vi "Operation_1600X900.vi"() -> ()   [LabVIEW 2015]
uses:
  Global/Globalclient.vi
panel:
  in  "F 4":bool
  in  "F 3":bool
  in  "F 2":bool
  in  "F 1":bool
  in  "Stop Button":bool
  out "删除通道":string[](array[string])
  out "选中行":i32
  in  "Tab":enum32{"用户管理", "通道控制", "通道监测", "温度&风扇"}(tab)=enum."通道控制"
  out "连接数":u8
  out "未登陆":string[][](table)=[["admin", "123456", "ADMIN"], ["api1", "333333", "API"], ["api2", "333333", "API"], ["api3", "333333", "API"], ["weily", "123", "GENERAL"]]
  out "已登陆":string[][](table)
  in  "Add Button":bool
  in  "Remove Button":bool
  out "删除用户":string
  out "时钟":string[][](table)
  out "射频":string[][](table)
  in  "查询开关":bool
  in  "释放所有":bool
  out "LOSS":cluster{dbl[], dbl[]}[](graph)
  in  "申请通道":bool
  in  "释放通道":bool
  in  "查询差损":bool
  in  "通道":i32[](listbox)
  in  "Tab":enum32{"RF", "CLK"}(tab)
  in  "监控":enum32{"RF", "TIME"}(tab)
  out "b 1":bool
  out "b 2":bool
  out "b 3":bool
  out "b 4":bool
  out "b 5":bool
  out "b 6":bool
  out "b 7":bool
  out "b 8":bool
  out "b 9":bool
  out "b 10":bool
  out "b 11":bool
  out "b 12":bool
  out "b 13":bool
  out "b 14":bool
  out "b 15":bool
  out "b 16":bool
  out "b 17":bool
  out "b 18":bool
  out "b 19":bool
  out "b 20":bool
  out "b 21":bool
  out "b 22":bool
  out "b 23":bool
  out "b 24":bool
  out "b 25":bool
  out "b 26":bool
  out "b 27":bool
  out "b 28":bool
  out "b 29":bool
  out "b 30":bool
  out "b 31":bool
  out "b 32":bool
  out "S 1":string
  out "S 2":string
  out "S 3":string
  out "S 4":string
  out "S 5":string
  out "S 6":string
  out "S 7":string
  out "S 8":string
  out "S 9":string
  out "S 10":string
  out "S 11":string
  out "S 12":string
  out "S 13":string
  out "S 14":string
  out "S 15":string
  out "S 16":string
  out "S 17":string
  out "S 18":string
  out "S 19":string
  out "S 20":string
  out "S 21":string
  out "S 22":string
  out "S 23":string
  out "S 24":string
  out "S 25":string
  out "S 26":string
  out "S 27":string
  out "S 28":string
  out "S 29":string
  out "S 30":string
  out "S 31":string
  out "S 32":string
  out "b 33":bool
  out "b 41":bool
  out "b 49":bool
  out "b 57":bool
  out "S 33":string
  out "S 41":string
  out "S 49":string
  out "S 57":string
  out "a 9":bool
  out "b 34":bool
  out "b 42":bool
  out "b 50":bool
  out "b 58":bool
  out "S 34":string
  out "S 42":string
  out "S 50":string
  out "S 58":string
  out "a 10":bool
  out "b 35":bool
  out "b 43":bool
  out "b 51":bool
  out "b 59":bool
  out "S 35":string
  out "S 43":string
  out "S 51":string
  out "S 59":string
  out "a 11":bool
  out "b 36":bool
  out "b 44":bool
  out "b 52":bool
  out "b 60":bool
  out "S 36":string
  out "S 44":string
  out "S 52":string
  out "S 60":string
  out "a 12":bool
  out "b 37":bool
  out "b 45":bool
  out "b 53":bool
  out "b 61":bool
  out "S 37":string
  out "S 45":string
  out "S 53":string
  out "S 61":string
  out "a 13":bool
  out "b 38":bool
  out "b 46":bool
  out "b 54":bool
  out "b 62":bool
  out "S 38":string
  out "S 46":string
  out "S 54":string
  out "S 62":string
  out "a 14":bool
  out "b 39":bool
  out "b 47":bool
  out "b 55":bool
  out "b 63":bool
  out "S 39":string
  out "S 47":string
  out "S 55":string
  out "S 63":string
  out "a 15":bool
  out "b 40":bool
  out "b 48":bool
  out "b 56":bool
  out "b 64":bool
  out "S 40":string
  out "S 48":string
  out "S 56":string
  out "S 64":string
  out "a 16":bool
  out "A 9":bool
  out "A 16":bool
  out "A 15":bool
  out "A 14":bool
  out "A 13":bool
  out "A 12":bool
  out "A 11":bool
  out "A 10":bool
  out "A 1":bool
  out "a 1":bool
  out "a 2":bool
  out "A 2":bool
  out "a 3":bool
  out "A 3":bool
  out "a 4":bool
  out "A 4":bool
  out "a 5":bool
  out "A 5":bool
  out "a 6":bool
  out "A 6":bool
  out "a 7":bool
  out "A 7":bool
  out "a 8":bool
  out "A 8":bool
  out "COM 1":bool
  out "com_1":bool
  out "com_2":bool
  out "COM 2":bool
  out "com_3":bool
  out "COM 3":bool
  out "com_4":bool
  out "COM 4":bool
  out "T 1":bool caption="1"
  out "T 2":bool caption="2"
  out "T 3":bool caption="3"
  out "T 4":bool caption="4"
  out "T 5":bool caption="5"
  out "T 6":bool caption="6"
  out "T 7":bool caption="7"
  out "T 8":bool caption="8"
  out "T 9":bool caption="9"
  out "T 10":bool caption="10"
  out "T 11":bool caption="11"
  out "T 12":bool caption="12"
  out "T 13":bool caption="13"
  out "T 14":bool caption="14"
  out "T 15":bool caption="15"
  out "T 16":bool caption="16"
  out "T 17":bool caption="17"
  out "T 18":bool caption="18"
  out "T 19":bool caption="19"
  out "T 20":bool caption="20"
  out "T 21":bool caption="21"
  out "T 22":bool caption="22"
  out "T 23":bool caption="23"
  out "T 24":bool caption="24"
  out "T 25":bool caption="25"
  out "T 26":bool caption="26"
  out "T 27":bool caption="27"
  out "T 28":bool caption="28"
  out "T 29":bool caption="29"
  out "T 30":bool caption="30"
  out "T 31":bool caption="31"
  out "T 32":bool caption="32"
  out "T 33":bool caption="33"
  out "T 34":bool caption="34"
  out "T 35":bool caption="35"
  out "T 36":bool caption="36"
  out "T 37":bool caption="37"
  out "T 38":bool caption="38"
  out "T 39":bool caption="39"
  out "T 40":bool caption="40"
  out "T 41":bool caption="41"
  out "T 42":bool caption="42"
  out "T 43":bool caption="43"
  out "T 44":bool caption="44"
  out "T 45":bool caption="45"
  out "T 46":bool caption="46"
  out "T 47":bool caption="47"
  out "T 48":bool caption="48"
  out "OUT 1":bool
  out "OUT 2":bool
  out "OUT 4":bool
  out "OUT 3":bool
  out "OUT 5":bool
  out "OUT 6":bool
  out "OUT 8":bool
  out "OUT 7":bool
  in  "Alarm":bool
  in  "风扇 4":string
  out "FS 4":u16(ring)
  in  "风扇 3":string
  out "FS 3":u16(ring)
  in  "风扇 2":string
  out "FS 2":u16(ring)
  in  "风扇 1":string
  out "FS 1":u16(ring)
  out "温度 8":dbl(slide)=50.0 scale=0.0..100.0 scale format="%0.1f"
  out "温度 7":dbl(slide)=50.0 scale=0.0..100.0 scale format="%0.1f"
  out "温度 6":dbl(slide)=50.0 scale=0.0..100.0 scale format="%0.1f"
  out "温度 5":dbl(slide)=50.0 scale=0.0..100.0 scale format="%0.1f"
  out "温度 4":dbl(slide)=50.0 scale=0.0..100.0 scale format="%0.1f"
  out "温度 3":dbl(slide)=50.0 scale=0.0..100.0 scale format="%0.1f"
  out "温度 2":dbl(slide)=50.0 scale=0.0..100.0 scale format="%0.1f"
  out "温度 1":dbl(slide)=50.0 scale=0.0..100.0 scale format="%0.1f"
  in  "机箱":T1(tab)
  # "LCBB多路开关矩阵"
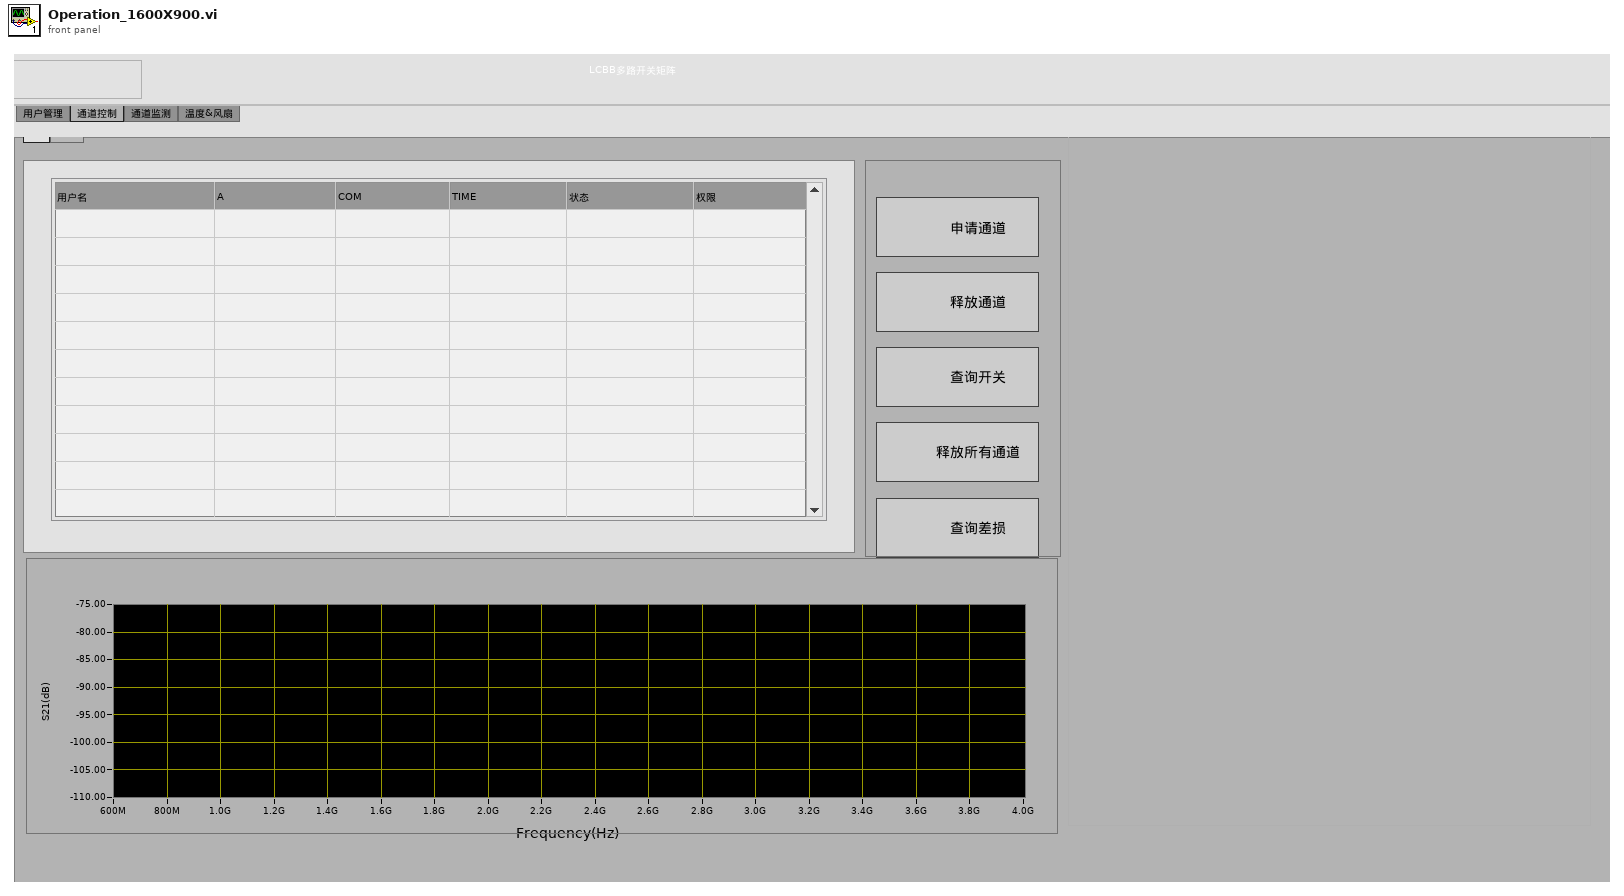
[diagram p1: front panel]
types:
  T1 = enum32{"机箱 1", "机箱 2", "机箱 3", "机箱 4", "机箱 5", "机箱 6", "机箱 7", "机箱 8", "主控 1", "机箱 9", "机箱 10", "机箱 11", "机箱 12", "机箱 13", "机箱 14", "机箱 15", "机箱 16", "主控 2"}
  T2 = enum16{"Standard", "Buffered", "CRLF", "Immediate"}
  T3 = typedef "LVPoint32TypeDef.ctl" = cluster{"Horizontal":i32, "Vertical":i32}
  T4 = typedef "LVRowAndColumnTypeDef.ctl" = cluster{"Row":i32, "Column":i32}
  T5 = cluster{"data name":string, "data data":string}[]
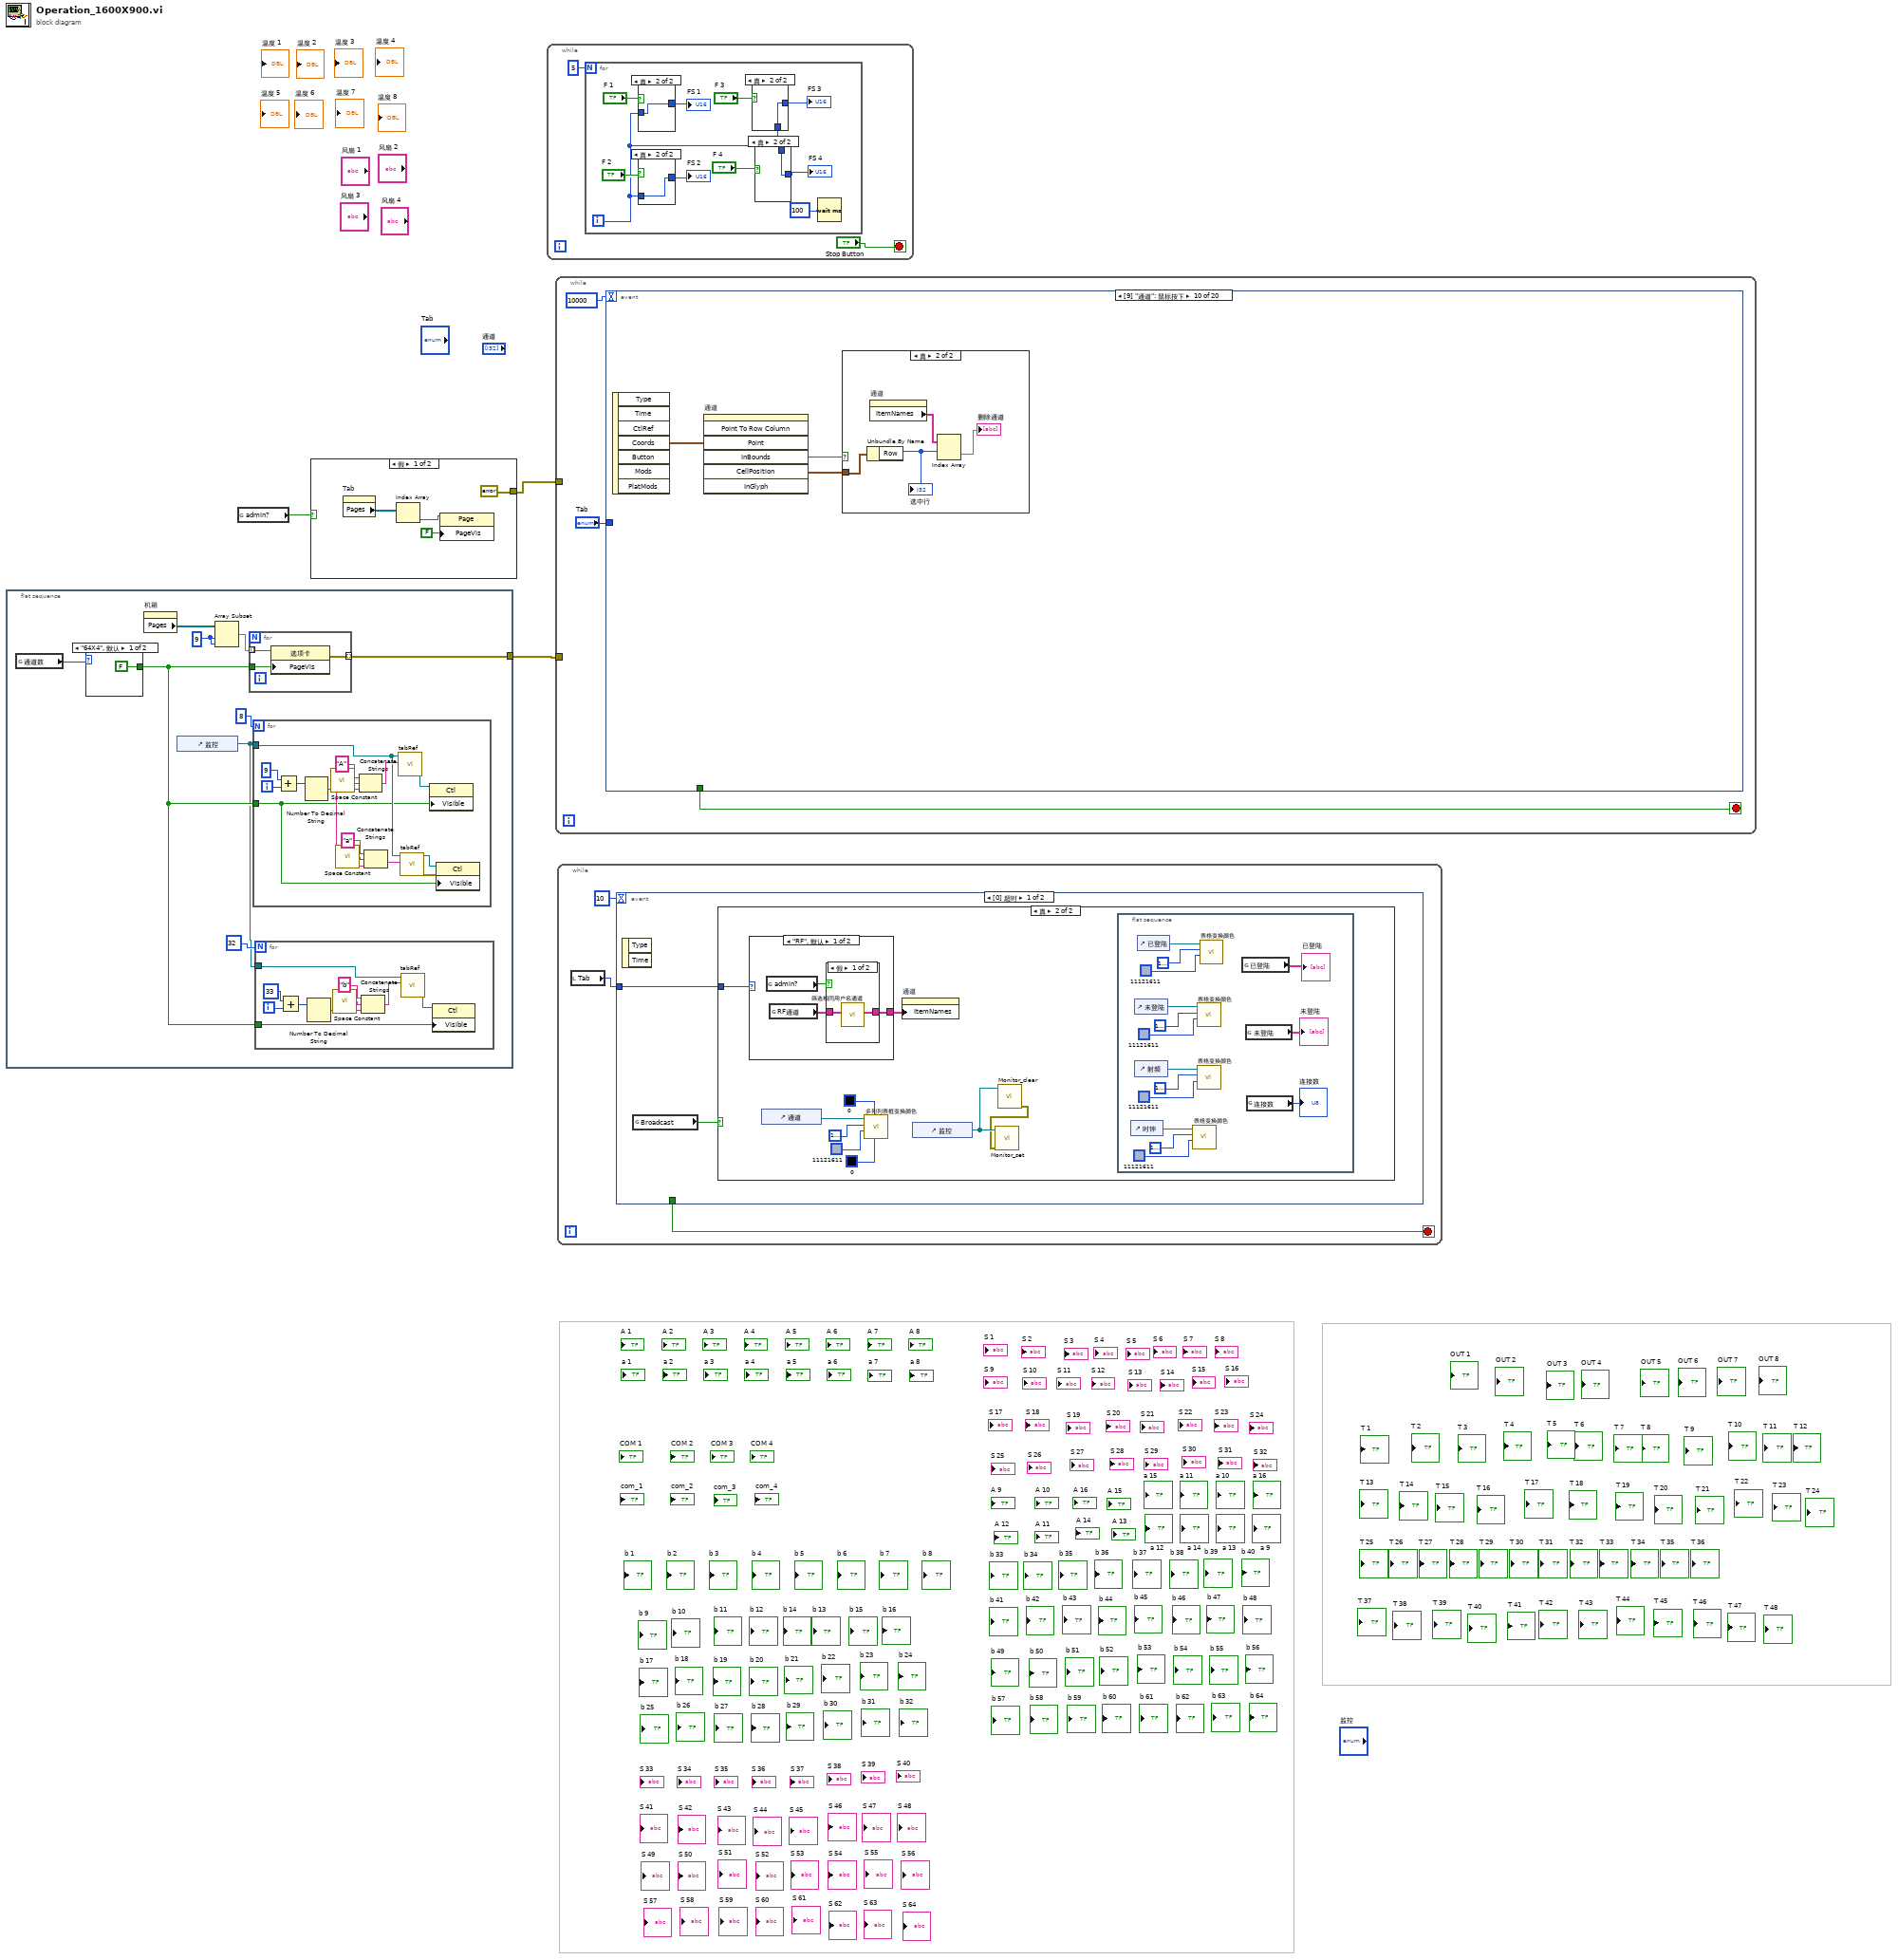
[diagram p0: block diagram]
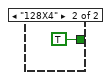
[diagram p2: hidden frame]
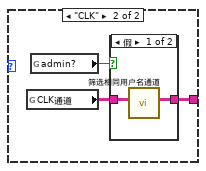
[diagram p5: hidden frame]
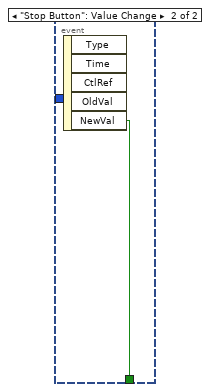
[diagram p7: hidden frame]
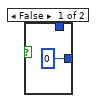
[diagram p8: hidden frame]
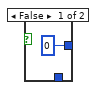
[diagram p9: hidden frame]
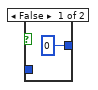
[diagram p10: hidden frame]
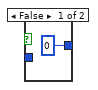
[diagram p11: hidden frame]
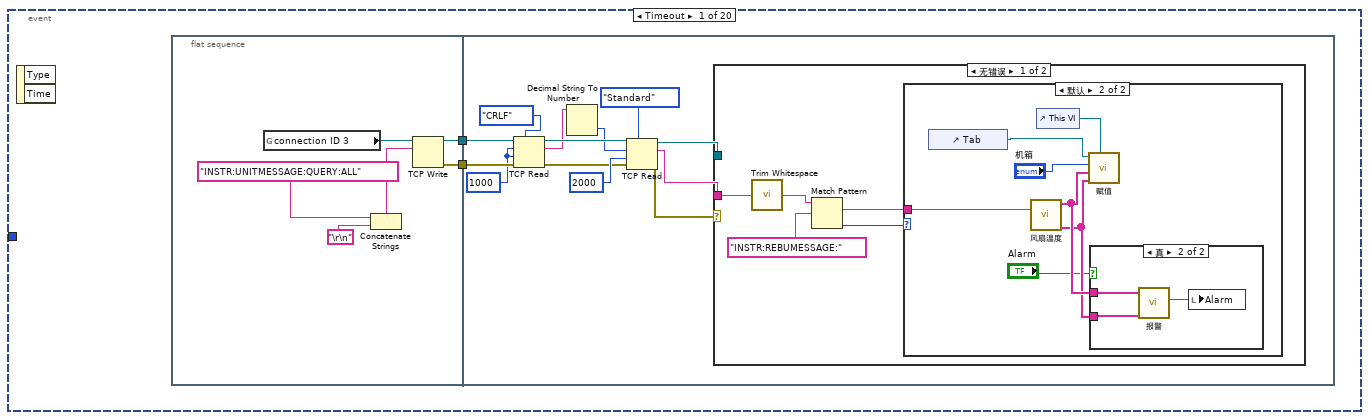
[diagram p13: hidden frame]
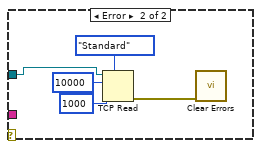
[diagram p16: hidden frame]
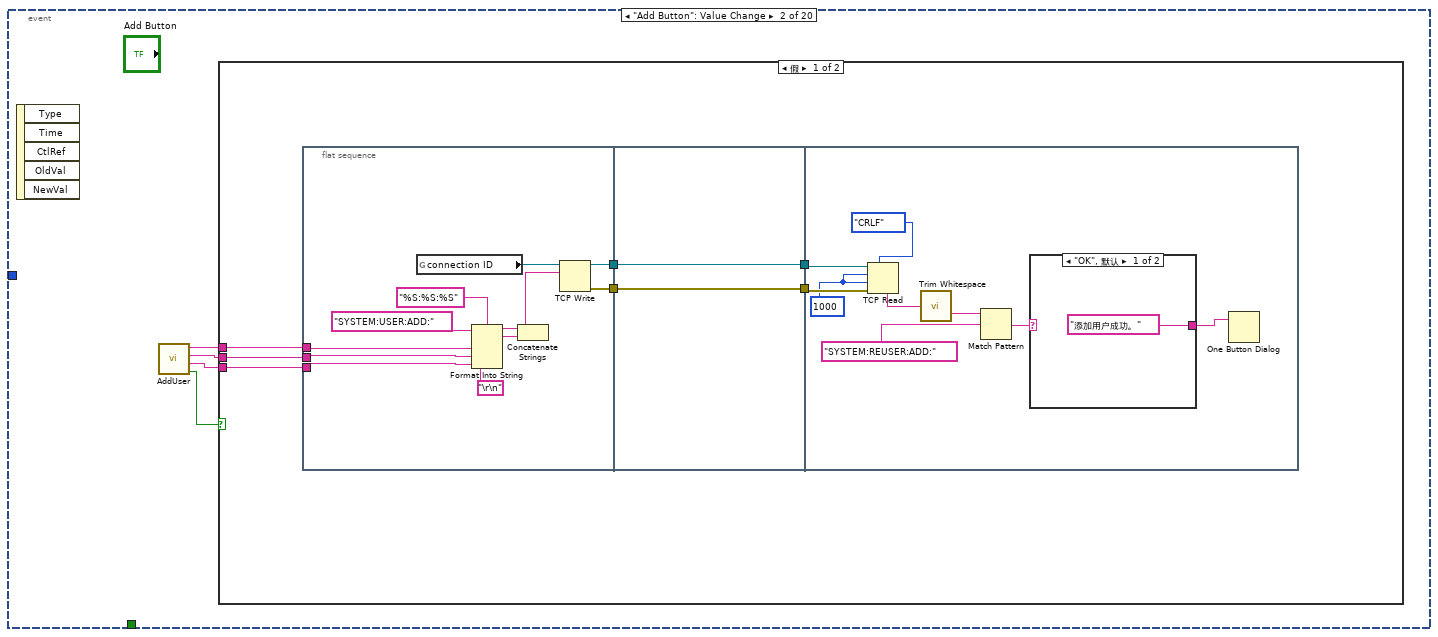
[diagram p17: hidden frame]
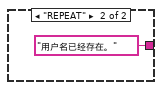
[diagram p18: hidden frame]
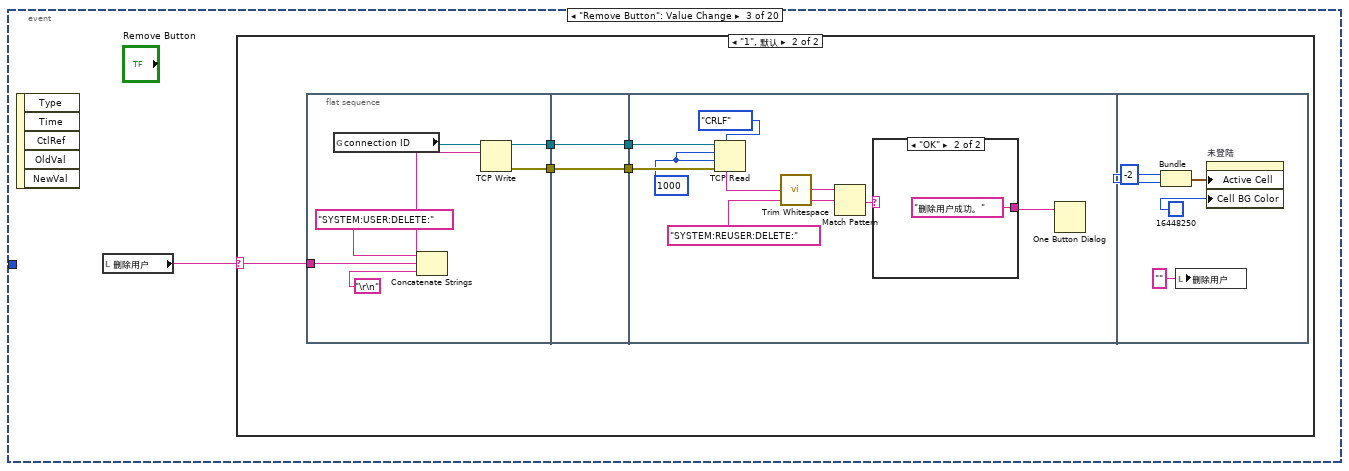
[diagram p20: hidden frame]
diagram:
  n1 = flat-sequence {
    tunnel: [w4] -> w1
    frame #0 {
      w10 = 9
      n2 = global read "Globalclient.vi" "通道数"() -> (w12:enum16{"64X4", "128X4"})
      n3 = case shown="\"64X4\", 默认" w12 {
        tunnel: [FALSE ("可见") TRUE ("可见")] -> w6
        frame "64X4", Default {
        }
        frame "128X4" {
        }
      }
      n4 = property on="机箱" class="TabCtl (严格)"() -> ("Pages"=w11:refnum<vi>[])  [unwired: 2 in, 2 out]
      n5 = control-ref of="监控"() -> (w5:refnum<vi>)
      n6 = Array Subset(array=w11, index=w10, length=w10) -> (w9:refnum<vi>[])
      n7 = for {
        tunnel: w9 -> [w40] mode=indexing
        tunnel: w6 -> [w39]
        tunnel: [w38] -> w4 mode=indexing
        n8 = property on="Property Node" class="选项卡"(reference=w40, "PageVis"=w39) -> (error out=w38:errorcluster)  [unwired: 1 in, 1 out]
      }
      n9 = for {
        N: 8 -> [_]
        tunnel: w6 -> [w23]
        tunnel: w5 -> [w26]
        i -> [w33]
        n10 = Add(x=9, y=w33) -> (x+y=w35:i32)
        n11 = Number To Decimal String(number=w35) -> (decimal integer string=w28:string)  [unwired: 1 in]
        n12 = call <vilib>:"Space Constant.vi"() -> ("String"=w37:string)
        n13 = call <vilib>:"Space Constant.vi"() -> ("String"=w29:string)
        n14 = Concatenate Strings("A" ("字符串"), w37, w28) -> (w32:string)
        n15 = Concatenate Strings("a" ("字符串"), w29, w28) -> (w27:string)
        n16 = call "tabRef.vi"("control name"=w32, "Tab Control"=w26) -> ("control refnum"=w31:refnum<vi>)  [unwired: 8 in, 1 out]
        n17 = call "tabRef.vi"("control name"=w27, "Tab Control"=w26) -> ("error out"=w24:errorcluster, "control refnum"=w25:refnum<vi>)  [unwired: 8 in]
        n18 = property class="Ctl"(reference=w31, "Visible"=w23) -> ()  [unwired: 1 in, 2 out]
        n19 = property class="Ctl"(reference=w25, error in=w24, "Visible"=w23) -> ()  [unwired: 2 out]
      }
      n20 = for {
        N: 32 -> [_]
        tunnel: w6 -> [w13]
        tunnel: w5 -> [w14]
        i -> [w18]
        n21 = Add(x=33, y=w18) -> (x+y=w20:i32)
        n22 = Number To Decimal String(number=w20) -> (decimal integer string=w15:string)  [unwired: 1 in]
        n23 = call <vilib>:"Space Constant.vi"() -> ("String"=w22:string)
        n24 = Concatenate Strings("b" ("字符串"), w22, w15) -> (w17:string)
        n25 = call "tabRef.vi"("control name"=w17, "Tab Control"=w14) -> ("control refnum"=w16:refnum<vi>)  [unwired: 8 in, 1 out]
        n26 = property class="Ctl"(reference=w16, "Visible"=w13) -> ()  [unwired: 1 in, 2 out]
      }
    }
  }
  n27 = global read "Globalclient.vi" "admin?"() -> (w3:bool)
  n28 = case shown="假" w3 {
    tunnel: [errorcluster {"status"=FALSE, "code"=0, "source"=""} ("error constant") _] -> w2
    frame False {
      n29 = property on="Tab" class="TabCtl (严格)"() -> ("Pages"=w46:refnum<vi>[])  [unwired: 2 in, 2 out]
      n30 = Index Array(array=w46) -> (element=w45:refnum<vi>)  [unwired: 1 in]
      n31 = property class="Page"(reference=w45, "PageVis"=FALSE ("Page Visible")) -> ()  [unwired: 1 in, 2 out]
    }
    frame True {
    }
  }
  n32 = while {
    stop <- "Stop Button" stop-if-true
    n33 = for {
      N: 5 -> [_]
      i -> [w50]
      n34 = case shown="真" "F 1" {
        tunnel: [0 w66] -> w57
        tunnel: w50 -> [_ w66]
        frame False {
        }
        frame True {
        }
      }
      "FS 1" <- w57
      n35 = case shown="真" "F 2" {
        tunnel: [0 w64] -> w55
        tunnel: w50 -> [_ w64]
        frame False {
        }
        frame True {
        }
      }
      "FS 2" <- w55
      n36 = case shown="真" "F 3" {
        tunnel: [0 w62] -> w54
        tunnel: w50 -> [_ w62]
        frame False {
        }
        frame True {
        }
      }
      "FS 3" <- w54
      n37 = case shown="真" "F 4" {
        tunnel: [0 w60] -> w51
        tunnel: w50 -> [_ w60]
        frame False {
        }
        frame True {
        }
      }
      "FS 4" <- w51
      n38 = Wait (ms)(milliseconds to wait=u32 100) -> ()  [unwired: 1 out]
    }
  }
  n39 = while {
    tunnel: w2 -> [_]
    tunnel: w1 -> [_]
    stop <- w69 stop-if-true
    n40 = event shown="[9] \"通道\": 鼠标按下" {
      selector: _ -> [_ _ _ _ _ _ _ _ _ _ _ _ _ _ _ _ _ _ _ _]
      dyn-events: _ -> [_ _ _ _ _ _ _ _ _ _ _ _ _ _ _ _ _ _ _ _]
      timeout: 10000 -> [_ _ _ _ _ _ _ _ _ _ _ _ _ _ _ _ _ _ _ _]
      tunnel: [_ _ _ _ _ _ _ _ _ _ _ _ _ _ _ _ _ _ _ w636] -> w69
      tunnel: "Tab" -> [_ _ _ _ _ w222 w261 w306 _ _ _ _ _ _ w433 _ _ _ _ _]
      event Timeout {
        n41 = event-data() -> ()  [unwired: 1 in, 2 out]
        n42 = flat-sequence {
          tunnel: [w74] -> w71
          tunnel: [w73] -> w70
          tunnel: w71 -> [w87]
          tunnel: w70 -> [w85]
          frame #0 {
            n43 = global read "Globalclient.vi" "connection ID 3"() -> (w77:refnum<k5>)
            n44 = Concatenate Strings("INSTR:UNITMESSAGE:QUERY:ALL", "\r\n") -> (w75:string)
            n45 = TCP Write(connection ID=w77, data in=w75) -> (connection ID out=w74:refnum<k5>, error out=w73:errorcluster)  [unwired: 2 in, 1 out]
          }
          frame #1 {
            w82 = u32 1000 ("milliseconds to wait")
            n46 = TCP Read(connection ID=w87, bytes to read=w82, error in (no error)=w85, 7:T2."CRLF" ("mode (standard)"), 9:w82) -> (connection ID out=w86:refnum<k5>, data out=w81:string, error out=w84:errorcluster)
            n47 = Decimal String To Number(string=w81) -> (number=w80:i32)  [unwired: 2 in, 1 out]
            n48 = TCP Read(connection ID=w86, bytes to read=w80, error in (no error)=w84, 7:T2."Standard" ("mode (standard)"), 9:u32 2000 ("milliseconds to wait")) -> (connection ID out=w78:refnum<k5>, data out=w88:string, error out=w79:errorcluster)
            n49 = case shown="无错误" w79 {
              tunnel: w88 -> [w95 _]
              tunnel: w78 -> [_ w110]
              frame No Error {
                n50 = call <vilib>:"Trim Whitespace.vi"("string"=w95) -> ("trimmed string"=w94:string)  [unwired: 1 in]
                n51 = Match Pattern(string=w94, regular expression="INSTR:REBUMESSAGE:") -> (after substring=w92:string, offset past match=w91:i32)  [unwired: 1 in, 2 out]
                n52 = case shown="默认" w91 {
                  tunnel: w92 -> [_ w102]
                  frame -1 {
                  }
                  frame Default {
                    n53 = control-ref of="Tab"() -> (w98:refnum<vi>)
                    n54 = call "风扇温度.vi"("order"=w102) -> ("temp"=w99:string[], "fengshan"=w100:string[])  [unwired: 9 in]
                    n55 = control-ref of="This VI"() -> (w101:refnum<vi>)
                    n56 = call "赋值.vi"("This VI"=w101, "temp"=w99, "fengshan"=w100, "机箱index"="机箱", "主控选项卡"=w98) -> ()  [unwired: 7 in]
                    n57 = case shown="真" "Alarm" {
                      tunnel: w100 -> [_ w105]
                      tunnel: w99 -> [_ w104]
                      frame False {
                      }
                      frame True {
                        n58 = call "报警.vi"("temp"=w104, "fengshan"=w105) -> ("ALARM"=w103:bool)  [unwired: 9 in]
                        n59 = local write "Alarm"(w103) -> ()
                      }
                    }
                  }
                }
              }
              frame Error {
                n60 = TCP Read(connection ID=w110, bytes to read=10000, 7:T2."Standard" ("mode (standard)"), 9:1000 ("timeout ms (25000)")) -> (error out=w106:errorcluster)  [unwired: 1 in, 2 out]
                n61 = call <vilib>:"Clear Errors.vi"("error in (no error)"=w106) -> ()  [unwired: 5 in, 2 out]
              }
            }
          }
        }
      }
      event "Add Button": Value Change {
        n62 = event-data() -> ()  [unwired: 1 in, 5 out]
        n63 = call "AddUser.vi"() -> ("drop?"=w111:bool, "Authority 2"=w114:string, "Password 2"=w113:string, "Username 2"=w112:string)  [unwired: 8 in]
        n64 = case shown="假" w111 {
          tunnel: w112 -> [w121 _]
          tunnel: w113 -> [w120 _]
          tunnel: w114 -> [w119 _]
          frame False {
            n65 = flat-sequence {
              tunnel: w121 -> [w129]
              tunnel: w120 -> [w128]
              tunnel: w119 -> [w127]
              tunnel: [w123] -> w117
              tunnel: [w122] -> w115
              tunnel: [w134] -> w118
              tunnel: w117 -> [w134]
              tunnel: [w133] -> w116
              tunnel: w115 -> [w133]
              tunnel: w118 -> [w143]
              tunnel: w116 -> [w142]
              frame #0 {
                n66 = global read "Globalclient.vi" "connection ID"() -> (w132:refnum<k5>)
                n67 = Format Into String(format string="%S:%S:%S", initial string="SYSTEM:USER:ADD:", w129, w128, w127) -> (resulting string=w126:string)  [unwired: 1 in, 1 out]
                n68 = Concatenate Strings(w126, "\r\n") -> (w124:string)
                n69 = TCP Write(connection ID=w132, data in=w124) -> (connection ID out=w123:refnum<k5>, error out=w122:errorcluster)  [unwired: 2 in, 1 out]
              }
              frame #1 {
              }
              frame #2 {
                w141 = u32 1000 ("milliseconds to wait")
                n70 = TCP Read(connection ID=w143, bytes to read=w141, error in (no error)=w142, 7:T2."CRLF" ("mode (standard)"), 9:w141) -> (data out=w139:string)  [unwired: 2 out]
                n71 = call <vilib>:"Trim Whitespace.vi"("string"=w139) -> ("trimmed string"=w138:string)  [unwired: 1 in]
                n72 = Match Pattern(string=w138, regular expression="SYSTEM:REUSER:ADD:") -> (after substring=w136:string)  [unwired: 1 in, 3 out]
                n73 = case shown="\"OK\", 默认" w136 {
                  tunnel: ["添加用户成功。" "用户名已经存在。"] -> w135
                  frame "OK", Default {
                  }
                  frame "REPEAT" {
                  }
                }
                n74 = One Button Dialog(message=w135) -> ()  [unwired: 1 in, 1 out]
              }
            }
          }
          frame True {
          }
        }
      }
      event "Remove Button": Value Change {
        n75 = event-data() -> ()  [unwired: 1 in, 5 out]
        n76 = local read "删除用户"() -> (w146:string)
        n77 = case shown="\"1\", 默认" w146 {
          selector: w146 -> [_ w152]
          frame "", "0" {
            n78 = One Button Dialog(message="请先选择未登陆表单中的一行。") -> ()  [unwired: 1 in, 1 out]
          }
          frame "1", Default {
            n79 = flat-sequence {
              tunnel: w152 -> [w156]
              tunnel: [w154] -> w150
              tunnel: [w153] -> w148
              tunnel: [w161] -> w151
              tunnel: w150 -> [w161]
              tunnel: [w160] -> w149
              tunnel: w148 -> [w160]
              tunnel: w151 -> [w170]
              tunnel: w149 -> [w169]
              frame #0 {
                n80 = global read "Globalclient.vi" "connection ID"() -> (w159:refnum<k5>)
                n81 = Concatenate Strings("SYSTEM:USER:DELETE:", w156, "\r\n") -> (w155:string)
                n82 = TCP Write(connection ID=w159, data in=w155) -> (connection ID out=w154:refnum<k5>, error out=w153:errorcluster)  [unwired: 2 in, 1 out]
              }
              frame #1 {
              }
              frame #2 {
                w167 = 1000
                n83 = TCP Read(connection ID=w170, bytes to read=w167, error in (no error)=w169, 7:T2."CRLF" ("mode (standard)"), 9:w167) -> (data out=w166:string)  [unwired: 2 out]
                n84 = call <vilib>:"Trim Whitespace.vi"("string"=w166) -> ("trimmed string"=w165:string)  [unwired: 1 in]
                n85 = Match Pattern(string=w165, regular expression="SYSTEM:REUSER:DELETE:") -> (after substring=w163:string)  [unwired: 1 in, 3 out]
                n86 = case shown="\"OK\"" w163 {
                  tunnel: ["删除用户失败。" "删除用户成功。"] -> w162
                  frame "False", Default {
                  }
                  frame "OK" {
                  }
                }
                n87 = One Button Dialog(message=w162) -> ()  [unwired: 1 in, 1 out]
              }
              frame #3 {
                w175 = -2 ("index")
                n88 = Bundle("index"=w175, "index"=w175) -> (w174:cluster{"index":i32, "index":i32})  [unwired: 1 in]
                n89 = local write "删除用户"("" ("删除用户")) -> ()
                n90 = property on="未登陆" class="Tbl (严格)"("Active Cell"=w174, "Cell BG Color"=u32 16448250) -> ()  [unwired: 2 in, 2 out]
              }
            }
          }
        }
      }
      event "未登陆": Mouse Down {
        n91 = event-data() -> ("Coords"=w177:T3)  [unwired: 1 in, 6 out]
        n92 = invoke on="未登陆" class="Tbl (strict)" method="Point To Row Column"("Point"=w177) -> ("InBounds"=w178:bool, "CellPosition"=w179:T4)  [unwired: 5 in, 4 out]
        n93 = case shown="真" w178 {
          tunnel: w179 -> [_ w185]
          frame False {
          }
          frame True {
            n94 = Unbundle By Name(w185) -> ("Row"=w180:i32)
            n95 = disable-structure shown="Disabled" {
              disable-tunnel: w180 -> [w186 _]
              frame Disabled {
                n96 = flat-sequence {
                  tunnel: w186 -> [w193]
                  frame #0 {
                    w189 = -2 ("index")
                    n97 = Bundle("index"=w189, "index"=w189) -> (w188:cluster{"index":i32, "index":i32})  [unwired: 1 in]
                    n98 = property on="未登陆" class="Tbl (严格)"("Active Cell"=w188, "Cell BG Color"=u32 16448250) -> ()  [unwired: 2 in, 2 out]
                  }
                  frame #1 {
                    n99 = Bundle("Row"=w193, "index"=-2) -> (w191:cluster{"Row":i32, "index":i32})  [unwired: 1 in]
                    n100 = property on="未登陆" class="Tbl (严格)"("Active Cell"=w191, "Cell BG Color"=u32 12369084) -> ()  [unwired: 2 in, 2 out]
                  }
                }
              }
              frame Enabled {
              }
            }
            n101 = property on="未登陆" class="Tbl (严格)"() -> ("Value"=w184:string[][])  [unwired: 2 in, 2 out]
            n102 = Index Array(array=w184, index (row)=w180) -> (element=w183:string[])  [unwired: 1 in]
            n103 = Index Array(array=w183, index=0) -> (element=→"删除用户":string)
          }
        }
      }
      event "已登陆": Mouse Down {
        n104 = event-data() -> ("Coords"=w194:T3)  [unwired: 1 in, 6 out]
        n105 = invoke on="已登陆" class="Tbl (strict)" method="Point To Row Column"("Point"=w194) -> ("InBounds"=w195:bool, "CellPosition"=w196:T4)  [unwired: 5 in, 4 out]
        n106 = case shown="真" w195 {
          tunnel: w196 -> [_ w217]
          frame False {
          }
          frame True {
            n107 = Unbundle By Name(w217) -> ("Row"=w215:i32)
            n108 = local read "已登陆"() -> (w216:string[][])
            n109 = global read "Globalclient.vi" "RF通道"() -> (w213:string[][])
            n110 = Index Array(array=w216, index (row)=w215, index (col)=0 ("disabled index (col)")) -> (element=w198:string)
            n111 = global read "Globalclient.vi" "CLK通道"() -> (w200:string[][])
            n112 = for {
              tunnel: w213 -> [w221] mode=indexing
              tunnel: [w220] -> w212 mode=indexing
              n113 = Index Array(array=w221) -> (element=w220:string)  [unwired: 1 in]
            }
            n114 = for {
              tunnel: w200 -> [w219] mode=indexing
              tunnel: [w218] -> w201 mode=indexing
              n115 = Index Array(array=w219) -> (element=w218:string)  [unwired: 1 in]
            }
            n116 = call <userlib>:"Search 1D Array (String)__ogtk.vi"("Array"=w212, "Element Data"=w198) -> ("Indices of Elements"=w211:i32[])  [unwired: 7 in]
            n117 = call <userlib>:"Search 1D Array (String)__ogtk.vi"("Array"=w201, "Element Data"=w198) -> ("Indices of Elements"=w202:i32[])  [unwired: 7 in]
            n118 = call <userlib>:"Delete Elements from 2D Array (String)__ogtk.vi"("delete (rows or columns)"=enum16{"rows", "columns"}."rows", "indices"=w211, "array"=w213) -> ("deleted elements"=w209:string[][])  [unwired: 7 in, 1 out]
            n119 = Array Subset(array=w209, index (col)=1 ("index"), length (col)=4 ("length")) -> (→"射频":string[][])  [unwired: 2 in]
            n120 = call <userlib>:"Delete Elements from 2D Array (String)__ogtk.vi"("delete (rows or columns)"=enum16{"rows", "columns"}."rows", "indices"=w202, "array"=w200) -> ("deleted elements"=w204:string[][])  [unwired: 7 in, 1 out]
            n121 = Array Subset(array=w204, index (col)=1 ("index"), length (col)=4 ("length")) -> (→"时钟":string[][])  [unwired: 2 in]
          }
        }
      }
      event "申请通道": Value Change {
        n122 = event-data() -> ()  [unwired: 1 in, 6 out]
        n123 = case shown="\"RF\", 默认" w222 {
          tunnel: [w230 w231] -> w226
          tunnel: [w229 w234] -> w225
          tunnel: [w228 w233] -> w224
          tunnel: [w227 w232] -> w223
          frame "RF", Default {
            n124 = call "ApplyRFdialog.vi"() -> ("drop?"=w230:bool, "时钟（分钟） 2"=w227:u32, "射频出 2"=w228:string, "射频进 2"=w229:string)  [unwired: 8 in]
          }
          frame "CLK" {
            n125 = call "ApplyCLKdialog.vi"() -> ("drop?"=w231:bool, "时间（分钟） 2"=w232:u32, "时钟出 2"=w233:string, "时钟进 2"=w234:string)  [unwired: 8 in]
          }
        }
        n126 = case shown="假" w226 {
          tunnel: w225 -> [w238 _]
          tunnel: w224 -> [w237 _]
          tunnel: w223 -> [w236 _]
          frame False {
            n127 = Format Into String(format string="%s:%s:%d", initial string="INSTR:ROUT:APPLY:", w238, w237, w236) -> (resulting string=w235:string)  [unwired: 1 in, 1 out]
            n128 = flat-sequence {
              tunnel: [w247] -> w244
              tunnel: [w246] -> w243
              tunnel: w235 -> [w245]
              tunnel: [w252] -> w242
              tunnel: w244 -> [w252]
              tunnel: [w251] -> w241
              tunnel: w243 -> [w251]
              tunnel: w242 -> [w260]
              tunnel: w241 -> [w259]
              frame #0 {
                n129 = global read "Globalclient.vi" "connection ID"() -> (w250:refnum<k5>)
                n130 = Concatenate Strings(w245, "\r\n") -> (w248:string)
                n131 = TCP Write(connection ID=w250, data in=w248) -> (connection ID out=w247:refnum<k5>, error out=w246:errorcluster)  [unwired: 2 in, 1 out]
              }
              frame #1 {
              }
              frame #2 {
                w257 = 1000
                n132 = TCP Read(connection ID=w260, bytes to read=w257, error in (no error)=w259, 7:T2."CRLF" ("mode (standard)"), 9:w257) -> (data out=w256:string)  [unwired: 2 out]
                n133 = call <vilib>:"Trim Whitespace.vi"("string"=w256) -> ("trimmed string"=w255:string)  [unwired: 1 in]
                n134 = Match Pattern(string=w255, regular expression="INSTR:REROUT:") -> (after substring=w253:string)  [unwired: 1 in, 3 out]
                n135 = case shown="\"False\", 默认" w253 {
                  frame "False", Default {
                  }
                  frame "NOW" {
                  }
                  frame "WAIT" {
                  }
                }
              }
            }
          }
          frame True {
          }
        }
      }
      event "释放通道": Value Change {
        n136 = event-data() -> ()  [unwired: 1 in, 6 out]
        n137 = local read "删除通道"() -> (w262:string[])
        n138 = Empty Array?(array=w262) -> (empty?=w263:bool)
        n139 = case shown="假" w263 {
          tunnel: w262 -> [w265 _]
          tunnel: w261 -> [w264 _]
          frame False {
            n140 = flat-sequence {
              tunnel: [w284] -> w269
              tunnel: [w283] -> w268
              tunnel: w265 -> [w277]
              tunnel: w264 -> [w270]
              tunnel: [w291] -> w267
              tunnel: w269 -> [w291]
              tunnel: [w290] -> w266
              tunnel: w268 -> [w290]
              tunnel: w267 -> [w299]
              tunnel: w266 -> [w298]
              frame #0 {
                n141 = case shown="\"RF\", 默认" w270 {
                  tunnel: ["A%s:COM%s:%s:%s" ("format string") "IN%s:OUT%s:%s:%s" ("format string")] -> w272
                  frame "RF", Default {
                  }
                  frame "CLK" {
                  }
                }
                n142 = Index Array(array=w277, index #1=1 ("index"), index #2=2 ("index"), index #3=0 ("index"), index #4=4 ("index")) -> (element #1=w276:string, element #2=w275:string, element #3=w274:string, element #4=w273:string)
                n143 = Format Into String(format string=w272, w276, w275, w274, w273) -> (resulting string=w271:string)  [unwired: 2 in, 1 out]
                n144 = global read "Globalclient.vi" "connection ID"() -> (w287:refnum<k5>)
                n145 = Concatenate Strings("INSTR:RELEASE:", w271, "\r\n") -> (w285:string)
                n146 = TCP Write(connection ID=w287, data in=w285) -> (connection ID out=w284:refnum<k5>, error out=w283:errorcluster)  [unwired: 2 in, 1 out]
              }
              frame #1 {
              }
              frame #2 {
                w296 = 1000
                n147 = TCP Read(connection ID=w299, bytes to read=w296, error in (no error)=w298, 7:T2."CRLF" ("mode (standard)"), 9:w296) -> (data out=w295:string)  [unwired: 2 out]
                n148 = call <vilib>:"Trim Whitespace.vi"("string"=w295) -> ("trimmed string"=w294:string)  [unwired: 1 in]
                n149 = Match Pattern(string=w294, regular expression="INSTR:RERELEASE:") -> (after substring=w292:string)  [unwired: 1 in, 3 out]
                n150 = case shown="\"NOW\"" w292 {
                  frame "False", Default {
                  }
                  frame "NOW" {
                  }
                  frame "WAIT" {
                  }
                }
              }
              frame #3 {
                n151 = local write "删除通道"(string[] [] ("删除通道")) -> ()
              }
            }
          }
          frame True {
            n152 = One Button Dialog(message="请先选择通道表单中的一行。") -> ()  [unwired: 1 in, 1 out]
          }
        }
      }
      event "释放所有": Value Change {
        n153 = event-data() -> ()  [unwired: 1 in, 6 out]
        n154 = flat-sequence {
          tunnel: [w311] -> w305
          tunnel: [w310] -> w304
          tunnel: w306 -> [w308]
          tunnel: [w318] -> w303
          tunnel: w305 -> [w318]
          tunnel: [w317] -> w302
          tunnel: w304 -> [w317]
          tunnel: w303 -> [w326]
          tunnel: w302 -> [w325]
          frame #0 {
            n155 = case shown="\"RF\", 默认" w308 {
              tunnel: ["RF" ("format string") "CLK" ("format string")] -> w307
              frame "RF", Default {
              }
              frame "CLK" {
              }
            }
            n156 = global read "Globalclient.vi" "connection ID"() -> (w314:refnum<k5>)
            n157 = Concatenate Strings("INSTR:RELEASEALL:", w307, "\r\n") -> (w312:string)
            n158 = TCP Write(connection ID=w314, data in=w312) -> (connection ID out=w311:refnum<k5>, error out=w310:errorcluster)  [unwired: 2 in, 1 out]
          }
          frame #1 {
          }
          frame #2 {
            w323 = 1000
            n159 = TCP Read(connection ID=w326, bytes to read=w323, error in (no error)=w325, 7:T2."CRLF" ("mode (standard)"), 9:w323) -> (data out=w322:string)  [unwired: 2 out]
            n160 = call <vilib>:"Trim Whitespace.vi"("string"=w322) -> ("trimmed string"=w321:string)  [unwired: 1 in]
            n161 = Match Pattern(string=w321, regular expression="INSTR:RERELEASEALL:") -> (after substring=w319:string)  [unwired: 1 in, 3 out]
            n162 = case shown="\"False\", 默认" w319 {
              frame "False", Default {
              }
              frame "NOW" {
              }
              frame "WAIT" {
              }
            }
          }
        }
      }
      event "查询差损": Value Change {
        n163 = event-data() -> ()  [unwired: 1 in, 6 out]
        n164 = call "QueryLossDialog.vi"() -> ("drop?"=w327:bool, "频率（KHz） 2"=w328:dbl, "射频出 2"=w329:string, "射频进 2"=w330:string)  [unwired: 8 in]
        n165 = case shown="假" w327 {
          tunnel: w330 -> [w337 _]
          tunnel: w329 -> [w336 _]
          tunnel: w328 -> [w335 _]
          frame False {
            n166 = Format Into String(format string="%s:%s:%.3f", initial string="INSTR:MANUALCAL:QUERY:", w337, w336, w335) -> (resulting string=w334:string)  [unwired: 1 in, 1 out]
            n167 = flat-sequence {
              tunnel: [w341] -> w332
              tunnel: [w340] -> w331
              tunnel: w334 -> [w339]
              tunnel: w332 -> [w359]
              tunnel: w331 -> [w358]
              frame #0 {
                n168 = global read "Globalclient.vi" "connection ID"() -> (w344:refnum<k5>)
                n169 = Concatenate Strings(w339, "\r\n") -> (w342:string)
                n170 = TCP Write(connection ID=w344, data in=w342) -> (connection ID out=w341:refnum<k5>, error out=w340:errorcluster)  [unwired: 2 in, 1 out]
              }
              frame #1 {
                w356 = 1000
                n171 = TCP Read(connection ID=w359, bytes to read=w356, error in (no error)=w358, 7:T2."CRLF" ("mode (standard)"), 9:w356) -> (data out=w355:string)  [unwired: 2 out]
                n172 = call <vilib>:"Trim Whitespace.vi"("string"=w355) -> ("trimmed string"=w354:string)  [unwired: 1 in]
                n173 = Match Pattern(string=w354, regular expression="INSTR:MANUALCAL:") -> (after substring=w352:string)  [unwired: 1 in, 3 out]
                n174 = call <userlib>:"String to 1D Array__ogtk.vi"("delimiter (Tab)"=":", "string"=w352) -> ("Array of Strings"=w350:string[])  [unwired: 9 in]
                n175 = Index Array(array=w350) -> (element #1=w348:string, element #2=w347:string, element #3=w346:string)  [unwired: 3 in]
                n176 = Format Into String(format string="%s%s的差损为：%s", w348, w347, w346) -> (resulting string=w345:string)  [unwired: 2 in, 1 out]
                n177 = One Button Dialog(message=w345) -> ()  [unwired: 1 in, 1 out]
              }
            }
          }
          frame True {
          }
        }
      }
      event "通道": Mouse Down {
        n178 = event-data() -> ("Coords"=w362:T3)  [unwired: 1 in, 6 out]
        n179 = invoke on="通道" class="MCListbox (strict)" method="Point To Row Column"("Point"=w362) -> ("InBounds"=w361:bool, "CellPosition"=w360:T4)  [unwired: 6 in, 5 out]
        n180 = case shown="真" w361 {
          tunnel: w360 -> [_ w366]
          frame False {
          }
          frame True {
            n181 = Unbundle By Name(w366) -> ("Row"=w365:i32)
            "选中行" <- w365
            n182 = property on="通道" class="MCListbox (严格)"() -> ("ItemNames"=w364:string[][])  [unwired: 2 in, 2 out]
            n183 = Index Array(array=w364, index (row)=w365) -> (element=→"删除通道":string[])  [unwired: 1 in]
          }
        }
      }
      event "Tab": Value Change {
        n184 = event-data() -> ("NewVal"=w369:enum32{"RF", "CLK"})  [unwired: 1 in, 4 out]
        n185 = case shown="\"CLK\"" w369 {
          tunnel: [string[] ["用户名", "A", "COM", "TIME", "状态", "权限", "", "", "", "", ""] ("Column Header Strings[]") string[] ["用户名", "IN", "OUT", "TIME", "状态", "权限", "", "", "", "", ""] ("Column Header Strings[]")] -> w368
          tunnel: [w370 w377] -> w367
          frame "RF", Default {
            n186 = global read "Globalclient.vi" "RF通道"() -> (w371:string[][])
            n187 = global read "Globalclient.vi" "admin?"() -> (w372:bool)
            n188 = case shown="假" w372 {
              tunnel: w371 -> [w375 w376]
              tunnel: [w374 w376] -> w370
              frame False {
                n189 = call "筛选相同用户名通道.vi"("通道in"=w375) -> ("通道"=w374:string[][])  [unwired: 10 in]
              }
              frame True {
              }
            }
          }
          frame "CLK" {
            n190 = global read "Globalclient.vi" "CLK通道"() -> (w378:string[][])
            n191 = global read "Globalclient.vi" "admin?"() -> (w379:bool)
            n192 = case shown="假" w379 {
              tunnel: w378 -> [w382 w383]
              tunnel: [w381 w383] -> w377
              frame False {
                n193 = call "筛选相同用户名通道.vi"("通道in"=w382) -> ("通道"=w381:string[][])  [unwired: 10 in]
              }
              frame True {
              }
            }
          }
        }
        n194 = property on="通道" class="MCListbox (严格)"("ColHdrString"=w368, "ItemNames"=w367) -> ()  [unwired: 2 in, 2 out]
      }
      event "通道": Drag Starting? {
        n195 = event-data() -> ()  [unwired: 1 in, 1 out]
        n196 = property on="通道" class="MCListbox (严格)"() -> ("ItemNames"=w393:string[][])  [unwired: 2 in, 2 out]
        n197 = local read "选中行"() -> (w392:i32)
        n198 = Index Array(array=w393, index (row)=w392) -> (element=w390:string[])  [unwired: 1 in]
        n199 = call <userlib>:"1D Array to String__ogtk.vi"("delimiter (Tab)"=":", "Array of Strings"=w390) -> ("delimited string"=w386:string)  [unwired: 9 in]
        n200 = Bundle By Name(cluster=cluster{"data name":string, "data data":string} {"data name"="", "data data"=""}, "data name"="SWMESSAGE", "data data"=w386) -> (w389:cluster{"data name":string, "data data":string})
        n201 = Build Array(w389) -> (w385:T5)
        n202 = event-data("Data"=w385, "Drag Mode"=enum32{"copy or move", "copy only", "move only"}."copy only") -> ()  [unwired: 1 in, 1 out]
      }
      event "查询开关": Value Change {
        n203 = event-data() -> ()  [unwired: 1 in, 5 out]
        n204 = call "QuerySwitchDialog.vi"() -> ("drop?"=w396:bool, "机箱选择 2"=w394:string, "开关箱编号 2"=w395:string)  [unwired: 9 in]
        n205 = case shown="假" w396 {
          tunnel: w395 -> [w398 _]
          tunnel: w394 -> [w400 _]
          frame False {
            n206 = Format Into String(format string="%s:%s", initial string="INSTR:SWMESSAGE:QUERY:", w398, w400) -> (resulting string=w402:string)  [unwired: 1 in, 1 out]
            n207 = flat-sequence {
              tunnel: [w410] -> w405
              tunnel: [w409] -> w404
              tunnel: w402 -> [w408]
              tunnel: w400 -> [w407]
              tunnel: [w407] -> w399
              tunnel: w398 -> [w406]
              tunnel: [w406] -> w397
              tunnel: w405 -> [w426]
              tunnel: w404 -> [w425]
              tunnel: w399 -> [w416]
              tunnel: w397 -> [w415]
              frame #0 {
                n208 = global read "Globalclient.vi" "connection ID"() -> (w413:refnum<k5>)
                n209 = Concatenate Strings(w408, "\r\n") -> (w411:string)
                n210 = TCP Write(connection ID=w413, data in=w411) -> (connection ID out=w410:refnum<k5>, error out=w409:errorcluster)  [unwired: 2 in, 1 out]
              }
              frame #1 {
                w423 = 1000
                n211 = TCP Read(connection ID=w426, bytes to read=w423, error in (no error)=w425, 7:T2."CRLF" ("mode (standard)"), 9:w423) -> (data out=w422:string)  [unwired: 2 out]
                n212 = call <vilib>:"Trim Whitespace.vi"("string"=w422) -> ("trimmed string"=w421:string)  [unwired: 1 in]
                n213 = Match Pattern(string=w421, regular expression="INSTR:RESWMESSAGE:") -> (after substring=w418:string)  [unwired: 1 in, 3 out]
                n214 = Match Pattern(string=w418, regular expression="SwitchTimes:") -> (after substring=w414:string, offset past match=w417:i32)  [unwired: 1 in, 2 out]
                n215 = case shown="1, 默认" w417 {
                  tunnel: w416 -> [_ w430]
                  tunnel: w415 -> [_ w429]
                  tunnel: w414 -> [_ w427]
                  frame -1 {
                  }
                  frame 1, Default {
                    n216 = Format Into String(format string="%s,%s号机箱的次数为：\n%s", w430, w429, w427) -> (resulting string=w428:string)  [unwired: 2 in, 1 out]
                    n217 = One Button Dialog(message=w428) -> ()  [unwired: 1 in, 1 out]
                  }
                }
              }
            }
          }
          frame True {
          }
        }
      }
      event "LOSS": Drag Enter {
        n218 = event-data() -> ()  [unwired: 1 in, 8 out]
        n219 = event-data("Accepted?"=TRUE) -> ()  [unwired: 1 in, 1 out]
      }
      event "LOSS": Drop {
        n220 = event-data() -> ()  [unwired: 1 in, 1 out]
        n221 = case shown="\"RF\", 默认" w433 {
          frame "RF", Default {
            n222 = Get Drag Drop Data(8:"" ("type"), 9:"SWMESSAGE" ("data name")) -> (3:w443:string)  [unwired: 1 in, 1 out]
            n223 = call <userlib>:"String to 1D Array__ogtk.vi"("delimiter (Tab)"=":", "string"=w443) -> ("Array of Strings"=w445:string[])  [unwired: 9 in]
            n224 = Index Array(array=w445, index #1=1 ("index"), index #2=2 ("index")) -> (element #1=w440:string, element #2=w439:string)
            n225 = Format Into String(format string="A%s:COM%s", initial string="INSTR:CALREAL:QUERY:", w440, w439) -> (resulting string=w438:string)  [unwired: 1 in, 1 out]
            n226 = flat-sequence {
              tunnel: [w452] -> w436
              tunnel: [w451] -> w435
              tunnel: w438 -> [w450]
              tunnel: w436 -> [w479]
              tunnel: w435 -> [w478]
              tunnel: [w468] -> w437
              frame #0 {
                n227 = global read "Globalclient.vi" "connection ID"() -> (w455:refnum<k5>)
                n228 = Concatenate Strings(w450, "\r\n") -> (w453:string)
                n229 = TCP Write(connection ID=w455, data in=w453) -> (connection ID out=w452:refnum<k5>, error out=w451:errorcluster)  [unwired: 2 in, 1 out]
              }
              frame #1 {
                n230 = TCP Read(connection ID=w479, bytes to read=102400, error in (no error)=w478, 7:T2."CRLF" ("mode (standard)"), 9:1000 ("timeout ms (25000)")) -> (data out=w475:string)  [unwired: 2 out]
                n231 = call <vilib>:"Trim Whitespace.vi"("string"=w475) -> ("trimmed string"=w474:string)  [unwired: 1 in]
                n232 = Match Pattern(string=w474, regular expression="INSTR:CALREAL:REQUERY:") -> (after substring=w470:string)  [unwired: 1 in, 3 out]
                n233 = call <userlib>:"String to 1D Array__ogtk.vi"("delimiter (Tab)"=":", "string"=w470) -> ("Array of Strings"=w471:string[])  [unwired: 9 in]
                n234 = Index Array(array=w471) -> (element #3=w466:string)  [unwired: 3 in, 2 out]
                n235 = call <userlib>:"String to 1D Array__ogtk.vi"("delimiter (Tab)"="$" ("search string"), "string"=w466) -> ("Array of Strings"=w464:string[])  [unwired: 9 in]
                n236 = Index Array(array=w464) -> (element #1=w463:string, element #2=w457:string)  [unwired: 2 in]
                n237 = call <userlib>:"String to 1D Array__ogtk.vi"("delimiter (Tab)"="&", "string"=w463) -> ("Array of Strings"=w461:string[])  [unwired: 9 in]
                n238 = call <userlib>:"String to 1D Array__ogtk.vi"("delimiter (Tab)"="&", "string"=w457) -> ("Array of Strings"=w459:string[])  [unwired: 9 in]
                n239 = Fract/Exp String To Number(string=w461) -> (number=w460:dbl[])  [unwired: 3 in, 1 out]
                n240 = Fract/Exp String To Number(string=w459) -> (number=w456:dbl[])  [unwired: 3 in, 1 out]
                n241 = Bundle(w460, w456) -> (w469:cluster{dbl[], dbl[]})  [unwired: 1 in]
                n242 = Build Array(w469) -> (w468:cluster{dbl[], dbl[]}[])
              }
            }
            "LOSS" <- w437
          }
          frame "CLK" {
          }
        }
        n243 = event-data("Accepted?"=TRUE) -> ()  [unwired: 1 in, 1 out]
      }
      event "b 1", "b 2", "b 3", "b 4", "b 5", "b 6", "b 7", "b 8", "b 9", "b 10", "b 11", "b 12", "b 13", "b 14", "b 15", "b 16", "b 17", "b 18", "b 19", "b 20", "b 21", "b 22", "b 23", "b 24", "b 25", "b 26", "b 27", "b 28", "b 29", "b 30", "b 31", "b 32", "b 33", "b 34", "b 35", "b 36", "b 37", "b 38", "b 39", "b 40", "b 41", "b 42", "b 43", "b 44", "b 45", "b 46", "b 47", "b 48", "b 49", "b 50", "b 51", "b 52", "b 53", "b 54", "b 55", "b 56", "b 57", "b 58", "b 59", "b 60", "b 61", "b 62", "b 63", "b 64": Shortcut Menu Activation? {
        n244 = event-data() -> ("MenuRef"=w481:refnum<k9>)  [unwired: 1 in, 5 out]
        n245 = global read "Globalclient.vi" "admin?"() -> (w480:bool)
        n246 = case shown="假" w480 {
          tunnel: [string[] ["WEILY_APPLY_CHANNEL", "APP_SEPARATOR", "WEILY_RELEASE_CHANNEL"] ("item tags") string[] ["WEILY_APPLY_CHANNEL"] ("item tags")] -> w483
          tunnel: [string[] ["APPLY_CHANNEL", "APP_SEPARATOR", "RELEASE_CHANNEL"] ("item names") string[] ["APPLY_CHANNEL"] ("item names")] -> w482
          frame True {
          }
          frame False {
          }
        }
        n247 = Delete Menu Items(9:w481) -> (3:w484:refnum<k9>)  [unwired: 3 in, 1 out]
        n248 = Insert Menu Items(7:w483, 8:w482, 9:w484) -> ()  [unwired: 3 in, 3 out]
        n249 = event-data() -> ()  [unwired: 2 in, 1 out]
      }
      event "b 1", "b 2", "b 3", "b 4", "b 5", "b 6", "b 7", "b 8", "b 9", "b 10", "b 11", "b 12", "b 13", "b 14", "b 15", "b 16", "b 17", "b 18", "b 19", "b 20", "b 21", "b 22", "b 23", "b 24", "b 25", "b 26", "b 27", "b 28", "b 29", "b 30", "b 31", "b 32", "b 33", "b 34", "b 35", "b 36", "b 37", "b 38", "b 39", "b 40", "b 41", "b 42", "b 43", "b 44", "b 45", "b 46", "b 47", "b 48", "b 49", "b 50", "b 51", "b 52", "b 53", "b 54", "b 55", "b 56", "b 57", "b 58", "b 59", "b 60", "b 61", "b 62", "b 63", "b 64": Shortcut Menu Selection (User) {
        n250 = event-data() -> ("CtlRef"=w489:refnum<vi>, "ItemTag"=w490:string)  [unwired: 1 in]
        n251 = case shown="\"WEILY_APPLY_CHANNEL\", 默认" w490 {
          tunnel: w489 -> [w495 w525]
          frame "WEILY_APPLY_CHANNEL", Default {
            n252 = call "ApplyRFdialog_2.vi"("CtlRef"=w495) -> ("drop?"=w492:bool, "时钟（分钟） 2"=w491:u32, "射频出"=w493:string, "射频进 2"=w494:string)  [unwired: 7 in]
            n253 = case shown="假" w492 {
              tunnel: w494 -> [w499 _]
              tunnel: w493 -> [w498 _]
              tunnel: w491 -> [w497 _]
              frame False {
                n254 = Format Into String(format string="%s:%s:%d", initial string="INSTR:ROUT:APPLY:", w499, w498, w497) -> (resulting string=w496:string)  [unwired: 1 in, 1 out]
                n255 = flat-sequence {
                  tunnel: [w508] -> w505
                  tunnel: [w507] -> w504
                  tunnel: w496 -> [w506]
                  tunnel: [w513] -> w503
                  tunnel: w505 -> [w513]
                  tunnel: [w512] -> w502
                  tunnel: w504 -> [w512]
                  tunnel: w503 -> [w521]
                  tunnel: w502 -> [w520]
                  frame #0 {
                    n256 = global read "Globalclient.vi" "connection ID"() -> (w511:refnum<k5>)
                    n257 = Concatenate Strings(w506, "\r\n") -> (w509:string)
                    n258 = TCP Write(connection ID=w511, data in=w509) -> (connection ID out=w508:refnum<k5>, error out=w507:errorcluster)  [unwired: 2 in, 1 out]
                  }
                  frame #1 {
                  }
                  frame #2 {
                    w518 = 1000
                    n259 = TCP Read(connection ID=w521, bytes to read=w518, error in (no error)=w520, 7:T2."CRLF" ("mode (standard)"), 9:w518) -> (data out=w517:string)  [unwired: 2 out]
                    n260 = call <vilib>:"Trim Whitespace.vi"("string"=w517) -> ("trimmed string"=w516:string)  [unwired: 1 in]
                    n261 = Match Pattern(string=w516, regular expression="INSTR:REROUT:") -> (after substring=w514:string)  [unwired: 1 in, 3 out]
                    n262 = case shown="\"False\", 默认" w514 {
                      frame "False", Default {
                      }
                      frame "NOW" {
                      }
                      frame "WAIT" {
                      }
                    }
                  }
                }
              }
              frame True {
              }
            }
          }
          frame "WEILY_RELEASE_CHANNEL" {
            n263 = global read "Globalclient.vi" "RF通道"() -> (w522:string[][])
            n264 = call "GetDeleteChannel.vi"("CHANNEL"=w522, "CtlRef"=w525) -> ("Finded"=w524:bool, "通道"=w523:string[])  [unwired: 8 in]
            n265 = case shown="真" w524 {
              tunnel: w523 -> [_ w526]
              frame False {
              }
              frame True {
                n266 = flat-sequence {
                  tunnel: [w544] -> w530
                  tunnel: [w543] -> w529
                  tunnel: w526 -> [w537]
                  tunnel: [w549] -> w528
                  tunnel: w530 -> [w549]
                  tunnel: [w548] -> w527
                  tunnel: w529 -> [w548]
                  tunnel: w528 -> [w557]
                  tunnel: w527 -> [w556]
                  frame #0 {
                    n267 = Index Array(array=w537, index #1=1 ("index"), index #2=2 ("index"), index #3=0 ("index"), index #4=4 ("index")) -> (element #1=w536:string, element #2=w535:string, element #3=w534:string, element #4=w533:string)
                    n268 = Format Into String(format string="A%s:COM%s:%s:%s", w536, w535, w534, w533) -> (resulting string=w531:string)  [unwired: 2 in, 1 out]
                    n269 = global read "Globalclient.vi" "connection ID"() -> (w547:refnum<k5>)
                    n270 = Concatenate Strings("INSTR:RELEASE:", w531, "\r\n") -> (w545:string)
                    n271 = TCP Write(connection ID=w547, data in=w545) -> (connection ID out=w544:refnum<k5>, error out=w543:errorcluster)  [unwired: 2 in, 1 out]
                  }
                  frame #1 {
                  }
                  frame #2 {
                    w554 = 1000
                    n272 = TCP Read(connection ID=w557, bytes to read=w554, error in (no error)=w556, 7:T2."CRLF" ("mode (standard)"), 9:w554) -> (data out=w553:string)  [unwired: 2 out]
                    n273 = call <vilib>:"Trim Whitespace.vi"("string"=w553) -> ("trimmed string"=w552:string)  [unwired: 1 in]
                    n274 = Match Pattern(string=w552, regular expression="INSTR:RERELEASE:") -> (after substring=w550:string)  [unwired: 1 in, 3 out]
                    n275 = case shown="\"NOW\"" w550 {
                      frame "False", Default {
                      }
                      frame "NOW" {
                      }
                      frame "WAIT" {
                      }
                    }
                  }
                }
              }
            }
          }
        }
      }
      event "T 1", "T 2", "T 3", "T 4", "T 5", "T 6", "T 7", "T 8", "T 9", "T 10", "T 11", "T 12", "T 13", "T 14", "T 15", "T 16", "T 17", "T 18", "T 19", "T 20", "T 21", "T 22", "T 23", "T 24", "T 25", "T 26", "T 27", "T 28", "T 29", "T 30", "T 31", "T 32", "T 33", "T 34", "T 35", "T 36", "T 37", "T 38", "T 39", "T 40", "T 41", "T 42", "T 43", "T 44", "T 45", "T 46", "T 47", "T 48": Shortcut Menu Activation? {
        n276 = event-data() -> ("MenuRef"=w561:refnum<k9>)  [unwired: 1 in, 3 out]
        n277 = global read "Globalclient.vi" "admin?"() -> (w560:bool)
        n278 = case shown="假" w560 {
          tunnel: [string[] ["WEILY_APPLY_CHANNEL", "APP_SEPARATOR", "WEILY_RELEASE_CHANNEL"] ("item tags") string[] ["WEILY_APPLY_CHANNEL"] ("item tags")] -> w558
          tunnel: [string[] ["APPLY_CHANNEL", "APP_SEPARATOR", "RELEASE_CHANNEL"] ("item names") string[] ["APPLY_CHANNEL"] ("item names")] -> w559
          frame True {
          }
          frame False {
          }
        }
        n279 = Delete Menu Items(9:w561) -> (3:w562:refnum<k9>)  [unwired: 3 in, 1 out]
        n280 = Insert Menu Items(7:w558, 8:w559, 9:w562) -> ()  [unwired: 3 in, 3 out]
        n281 = event-data() -> ()  [unwired: 2 in, 1 out]
      }
      event "T 1", "T 2", "T 3", "T 4", "T 5", "T 6", "T 7", "T 8", "T 9", "T 10", "T 11", "T 12", "T 13", "T 14", "T 15", "T 16", "T 17", "T 18", "T 19", "T 20", "T 21", "T 22", "T 23", "T 24", "T 25", "T 26", "T 27", "T 28", "T 29", "T 30", "T 31", "T 32", "T 33", "T 34", "T 35", "T 36", "T 37", "T 38", "T 39", "T 40", "T 41", "T 42", "T 43", "T 44", "T 45", "T 46", "T 47", "T 48": Shortcut Menu Selection (User) {
        n282 = event-data() -> ("CtlRef"=w567:refnum<vi>, "ItemTag"=w568:string)  [unwired: 1 in, 3 out]
        n283 = case shown="\"WEILY_APPLY_CHANNEL\", 默认" w568 {
          tunnel: w567 -> [w572 w609]
          frame "WEILY_RELEASE_CHANNEL" {
            n284 = global read "Globalclient.vi" "CLK通道"() -> (w571:string[][])
            n285 = call "GetDeleteChannel_CLK.vi"("CHANNEL"=w571, "CtlRef"=w572) -> ("Finded"=w569:bool, "通道"=w570:string[])  [unwired: 8 in]
            n286 = case shown="真" w569 {
              tunnel: w570 -> [_ w573]
              frame False {
              }
              frame True {
                n287 = flat-sequence {
                  tunnel: [w591] -> w577
                  tunnel: [w590] -> w576
                  tunnel: w573 -> [w584]
                  tunnel: [w596] -> w575
                  tunnel: w577 -> [w596]
                  tunnel: [w595] -> w574
                  tunnel: w576 -> [w595]
                  tunnel: w575 -> [w604]
                  tunnel: w574 -> [w603]
                  frame #0 {
                    n288 = Index Array(array=w584, index #1=1 ("index"), index #2=2 ("index"), index #3=0 ("index"), index #4=4 ("index")) -> (element #1=w583:string, element #2=w582:string, element #3=w581:string, element #4=w580:string)
                    n289 = Format Into String(format string="IN%s:OUT%s:%s:%s", w583, w582, w581, w580) -> (resulting string=w578:string)  [unwired: 2 in, 1 out]
                    n290 = global read "Globalclient.vi" "connection ID"() -> (w594:refnum<k5>)
                    n291 = Concatenate Strings("INSTR:RELEASE:", w578, "\r\n") -> (w592:string)
                    n292 = TCP Write(connection ID=w594, data in=w592) -> (connection ID out=w591:refnum<k5>, error out=w590:errorcluster)  [unwired: 2 in, 1 out]
                  }
                  frame #1 {
                  }
                  frame #2 {
                    w601 = 1000
                    n293 = TCP Read(connection ID=w604, bytes to read=w601, error in (no error)=w603, 7:T2."CRLF" ("mode (standard)"), 9:w601) -> (data out=w600:string)  [unwired: 2 out]
                    n294 = call <vilib>:"Trim Whitespace.vi"("string"=w600) -> ("trimmed string"=w599:string)  [unwired: 1 in]
                    n295 = Match Pattern(string=w599, regular expression="INSTR:RERELEASE:") -> (after substring=w597:string)  [unwired: 1 in, 3 out]
                    n296 = case shown="\"False\", 默认" w597 {
                      frame "False", Default {
                      }
                      frame "NOW" {
                      }
                      frame "WAIT" {
                      }
                    }
                  }
                }
              }
            }
          }
          frame "WEILY_APPLY_CHANNEL", Default {
            n297 = call "ApplyCLKdialog_2.vi"("CtlRef"=w609) -> ("drop?"=w608:bool, "时间（分钟） 2"=w605:u32, "时钟出 2"=w606:string, "时钟进"=w607:string)  [unwired: 7 in]
            n298 = case shown="假" w608 {
              tunnel: w607 -> [w612 _]
              tunnel: w606 -> [w611 _]
              tunnel: w605 -> [w610 _]
              frame False {
                n299 = Format Into String(format string="%s:%s:%d", initial string="INSTR:ROUT:APPLY:", w612, w611, w610) -> (resulting string=w613:string)  [unwired: 1 in, 1 out]
                n300 = flat-sequence {
                  tunnel: [w622] -> w619
                  tunnel: [w621] -> w618
                  tunnel: w613 -> [w620]
                  tunnel: [w627] -> w617
                  tunnel: w619 -> [w627]
                  tunnel: [w626] -> w616
                  tunnel: w618 -> [w626]
                  tunnel: w617 -> [w635]
                  tunnel: w616 -> [w634]
                  frame #0 {
                    n301 = global read "Globalclient.vi" "connection ID"() -> (w625:refnum<k5>)
                    n302 = Concatenate Strings(w620, "\r\n") -> (w623:string)
                    n303 = TCP Write(connection ID=w625, data in=w623) -> (connection ID out=w622:refnum<k5>, error out=w621:errorcluster)  [unwired: 2 in, 1 out]
                  }
                  frame #1 {
                  }
                  frame #2 {
                    w632 = 1000
                    n304 = TCP Read(connection ID=w635, bytes to read=w632, error in (no error)=w634, 7:T2."CRLF" ("mode (standard)"), 9:w632) -> (data out=w631:string)  [unwired: 2 out]
                    n305 = call <vilib>:"Trim Whitespace.vi"("string"=w631) -> ("trimmed string"=w630:string)  [unwired: 1 in]
                    n306 = Match Pattern(string=w630, regular expression="INSTR:REROUT:") -> (after substring=w628:string)  [unwired: 1 in, 3 out]
                    n307 = case shown="\"False\", 默认" w628 {
                      frame "False", Default {
                      }
                      frame "NOW" {
                      }
                      frame "WAIT" {
                      }
                    }
                  }
                }
              }
              frame True {
              }
            }
          }
        }
      }
      event "Stop Button": Value Change {
        n308 = event-data() -> ("NewVal"=w636:bool)  [unwired: 1 in, 4 out]
      }
    }
  }
  n309 = while {
    stop <- w637 stop-if-true
    n310 = local read "Tab"() -> (w638:enum32{"RF", "CLK"})
    n311 = event shown="[0] 超时" {
      selector: _ -> [_ _]
      dyn-events: _ -> [_ _]
      timeout: 10 -> [_ _]
      tunnel: w638 -> [w640 _]
      tunnel: [_ w678] -> w637
      event Timeout {
        n312 = event-data() -> ()  [unwired: 1 in, 2 out]
        n313 = global read "Globalclient.vi" "Broadcast"() -> (w641:bool)
        n314 = case shown="真" w641 {
          tunnel: w640 -> [_ w649]
          frame False {
          }
          frame True {
            n315 = case shown="\"RF\", 默认" w649 {
              tunnel: [w667 w672] -> w650
              frame "RF", Default {
                n316 = global read "Globalclient.vi" "admin?"() -> (w666:bool)
                n317 = global read "Globalclient.vi" "RF通道"() -> (w668:string[][])
                n318 = case shown="假" w666 {
                  tunnel: w668 -> [w670 w671]
                  tunnel: [w669 w671] -> w667
                  frame False {
                    n319 = call "筛选相同用户名通道.vi"("通道in"=w670) -> ("通道"=w669:string[][])  [unwired: 10 in]
                  }
                  frame True {
                  }
                }
              }
              frame "CLK" {
                n320 = global read "Globalclient.vi" "CLK通道"() -> (w673:string[][])
                n321 = global read "Globalclient.vi" "admin?"() -> (w674:bool)
                n322 = case shown="假" w674 {
                  tunnel: w673 -> [w676 w677]
                  tunnel: [w675 w677] -> w672
                  frame False {
                    n323 = call "筛选相同用户名通道.vi"("通道in"=w676) -> ("通道"=w675:string[][])  [unwired: 10 in]
                  }
                  frame True {
                  }
                }
              }
            }
            n324 = control-ref of="通道"() -> (w644:refnum<vi>)
            n325 = call "多列列表框变换颜色.vi"("奇数行字体颜色"=u32 0, "偶数行字体颜色"=u32 0, "奇数行背景颜色"=u32 11121611, "偶数行背景颜色"=u32 16777238, "MCListbox Refnum in"=w644) -> ()  [unwired: 5 in, 2 out]
            n326 = property on="通道" class="MCListbox (严格)"("ItemNames"=w650) -> ()  [unwired: 2 in, 2 out]
            n327 = control-ref of="监控"() -> (w643:refnum<vi>)
            n328 = call "Monitor_clear.vi"("Tab Control"=w643) -> ("error out"=w642:errorcluster)  [unwired: 10 in]
            n329 = call "Monitor_set.vi"("error in"=w642, "Tab Control"=w643) -> ()  [unwired: 9 in, 1 out]
            n330 = flat-sequence {
              frame #0 {
                n331 = control-ref of="时钟"() -> (w661:refnum<vi>)
                n332 = control-ref of="未登陆"() -> (w655:refnum<vi>)
                n333 = control-ref of="射频"() -> (w656:refnum<vi>)
                n334 = control-ref of="已登陆"() -> (w665:refnum<vi>)
                n335 = call "表格变换颜色.vi"("奇数行背景颜色"=u32 11121611, "偶数行背景颜色"=u32 16777238, "MCListbox Refnum in"=w661) -> ()  [unwired: 7 in, 2 out]
                n336 = call "表格变换颜色.vi"("奇数行背景颜色"=u32 11121611, "偶数行背景颜色"=u32 16777238, "MCListbox Refnum in"=w655) -> ()  [unwired: 7 in, 2 out]
                n337 = call "表格变换颜色.vi"("奇数行背景颜色"=u32 11121611, "偶数行背景颜色"=u32 16777238, "MCListbox Refnum in"=w656) -> ()  [unwired: 7 in, 2 out]
                n338 = call "表格变换颜色.vi"("奇数行背景颜色"=u32 11121611, "偶数行背景颜色"=u32 16777238, "MCListbox Refnum in"=w665) -> ()  [unwired: 7 in, 2 out]
                n339 = global read "Globalclient.vi" "已登陆"() -> (→"已登陆":string[][])
                n340 = global read "Globalclient.vi" "未登陆"() -> (→"未登陆":string[][])
                n341 = global read "Globalclient.vi" "连接数"() -> (→"连接数":i32)
              }
            }
          }
        }
      }
      event "Stop Button": Value Change {
        n342 = event-data() -> ("NewVal"=w678:bool)  [unwired: 1 in, 4 out]
      }
    }
  }
